vi "Lock in Amplifier.vi"() -> ()   [LabVIEW 2020]
uses:
  <vilib>/Utility/file.llb/Write Delimited Spreadsheet (DBL).vi
  Downloads/stanford_research_830/Stanford Research 830/Stanford Research 830.lvlib
panel:
  out "Waveform Graph":dynamicdata(graph)
  in  "Maximum Time (10000 ms)":u32=10000
  in  "Internal Reference Frequency (1000 Hz)":dbl=1000.0
  in  "Sine Output Amplitude (1 V)":dbl=1.0
  out "error out 2":errorcluster
  out "Measurements":sgl[](array[numeric])
  in  "Data Collection":T1={"Sample Rate (0: 62.5 mHz)"=0, "Continuous Storage (T: Enable)"=TRUE, "Number of Points (100)"=100, "Channel (1: Channel 1 Display)"=1, "Channel 1 Display (0: X)"=0} {"Channel 1 Display (0: X)" items=["X", "R", "X Noise", "Aux In 1", "Aux In 2"]; "Channel (1: Channel 1 Display)" items=["Channel 1 Display"=1, "Channel 2 Display"=2]; "Sample Rate (0: 62.5 mHz)" items=["62.5 mHz", "125 mHz", "250 mHz", "500 mHz", "1 Hz", "2 Hz", "4 Hz", "8Hz", "16 Hz", "32 Hz", "64 Hz", "128 Hz", "256 Hz", "512 Hz", "Trigger "]}
  in  "Configure":T2={"Lock in Amplifier PORT"="", "Input Connection (0: Single-Ended Voltage) "=0, "Input Coupling (0: AC)"=0, "Input Notch Filter (0: None)"=0, "Reference Source (1: Internal)"=1, "Dynamic Reserve (-1: Auto Reserve)"=-1, "Sensitivity (-1: Auto gain)"=-1, "Time Constant (8: 100ms)"=8} {"Time Constant (8: 100ms)" items=["10 us", "30 us", "100 us", "300 us", "1 ms", "3 ms", "10 ms", "30 ms", "100 ms", "300 ms", "1 s", "3 s", "10 s", "30 s", "100 s", "300 s", "1 ks", "3 ks", "10 ks", "30 ks"]; "Sensitivity (-1: Auto gain)" items=["Auto Gain"=-1, "2 nV/fA"=0, "5 nV/fA"=1, "10 nV/fA"=2, "20 nV/fA"=3, "50 nV/fA"=4, "100 nV/fA"=5, "200 nV/fA"=6, "500 nV/fA"=7, "1 uV/pA"=8, "2 uV/pA"=9, "5 uV/pA"=10, "10 uV/pA"=11, "20 uV/pA"=12, "50 uV/pA"=13, "100 uV/pA"=14, "200 uV/pA"=15, "500 uV/pA"=16, "1 mV/nA"=17, "2 mV/nA"=18, "5 mV/nA"=19, "10 mV/nA"=20, "20 mV/nA"=21, "50 mV/nA"=22, "100 mV/nA"=23, "200 mV/nA"=24, "500 mV/mA"=25, "1 V/uA"=26]; "Dynamic Reserve (-1: Auto Reserve)" items=["Auto Reserve"=-1, "High Reserve"=0, "Normal"=1, "Low Noise"=2]; "Reference Source (1: Internal)" items=["External", "Internal"]; "Input Notch Filter (0: None)" items=["None", "Line Notch", "2x Line Notch", "Both Notch Filters"]; "Input Coupling (0: AC)" items=["AC", "DC"]; "Input Connection (0: Single-Ended Voltage)" items=["Single-Ended Voltage", "Differential Voltage", "1 MOhm Current Gain", "100 MOhm Current Gain"]}
  out "error out":errorcluster
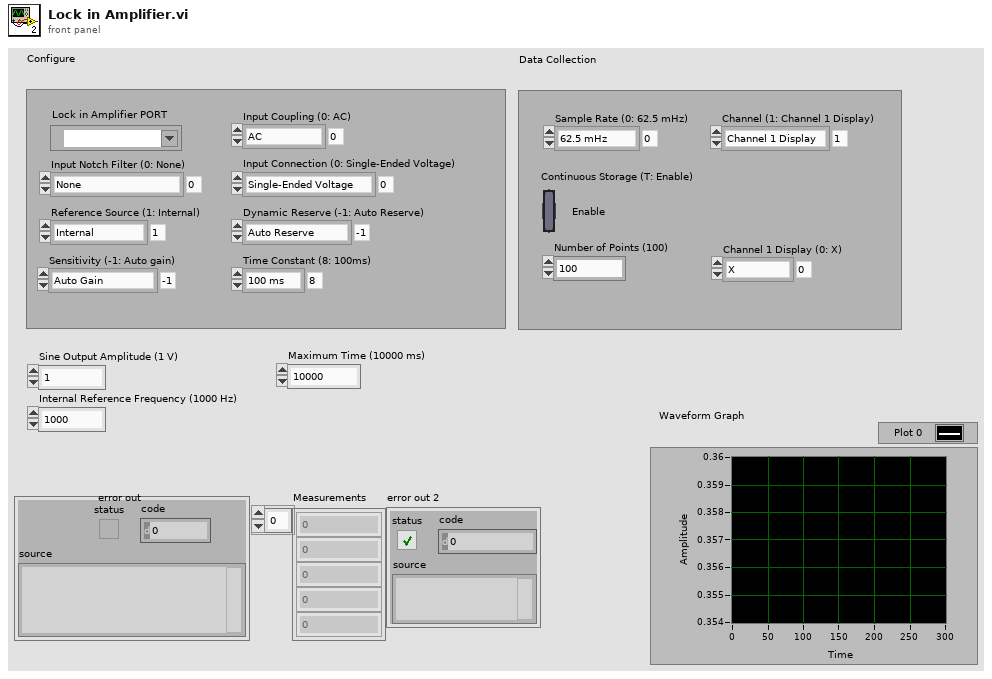
[diagram p1: front panel]
types:
  T1 = cluster{"Sample Rate (0: 62.5 mHz)":u16, "Continuous Storage (T: Enable)":bool, "Number of Points (100)":u32, "Channel (1: Channel 1 Display)":u16, "Channel 1 Display (0: X)":u16}
  T2 = cluster{"Lock in Amplifier PORT":refnum<visa-resource-name>, "Input Connection (0: Single-Ended Voltage) ":u16, "Input Coupling (0: AC)":u16, "Input Notch Filter (0: None)":u16, "Reference Source (1: Internal)":u16, "Dynamic Reserve (-1: Auto Reserve)":i16, "Sensitivity (-1: Auto gain)":i16, "Time Constant (8: 100ms)":u16}
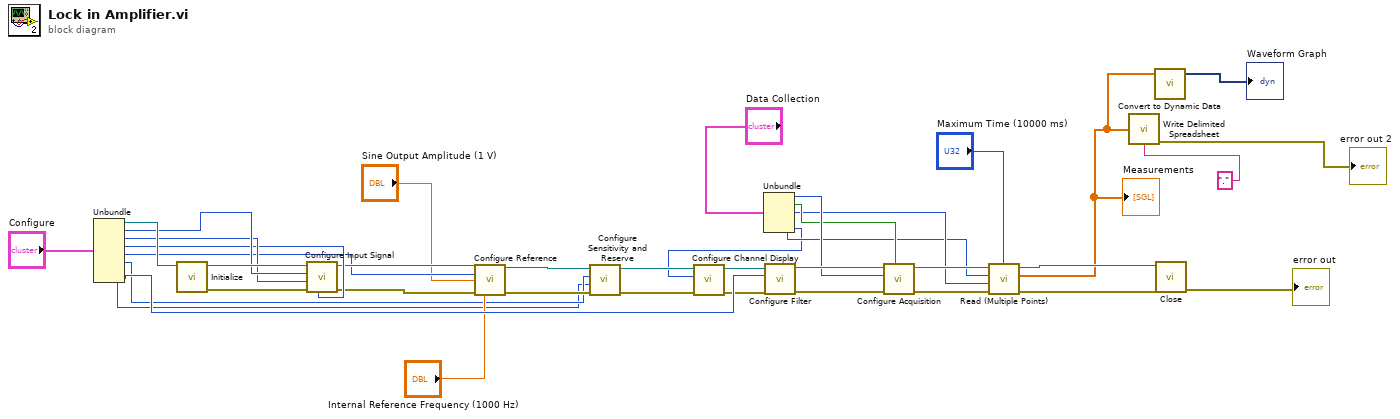
[diagram p0: block diagram]
diagram:
  n1 = Unbundle("Configure") -> ("Lock in Amplifier PORT"=w36:refnum<visa-resource-name>, "Input Connection (0: Single-Ended Voltage)"=w35:u16, "Input Coupling (0: AC)"=w34:u16, "Input Notch Filter (0: None)"=w33:u16, "Reference Source (1: Internal)"=w27:u16, "Dynamic Reserve (-1: Auto Reserve)"=w7:i16, "Sensitivity (-1: Auto gain)"=w6:i16, "Time Constant (8: 100ms)"=w25:u16)
  n2 = call "Initialize.vi"("VISA resource name"=w36) -> ("error out"=w38:errorcluster, "VISA resource name out"=w39:refnum<visa-resource-name>)  [unwired: 9 in]
  n3 = call "Configure Input Signal.vi"("Input Notch Filter (0: None)"=w33, "error in (no error)"=w38, "Input Coupling (0: AC)"=w34, "Input Connection (0: Single-Ended Voltage)"=w35, "VISA resource name"=w39) -> ("error out"=w26:errorcluster, "VISA resource name out"=w30:refnum<visa-resource-name>)  [unwired: 5 in]
  n4 = call "Configure Reference.vi"("VISA resource name"=w30, "Reference Source (1: Internal)"=w27, "Sine Output Amplitude (1 V)"="Sine Output Amplitude (1 V)", "error in (no error)"=w26, "Internal Reference Frequency (1000 Hz)"="Internal Reference Frequency (1000 Hz)") -> ("VISA resource name out"=w29:refnum<visa-resource-name>, "error out"=w28:errorcluster)  [unwired: 9 in]
  n5 = call "Configure Sensitivity and Reserve.vi"("error in (no error)"=w28, "Sensitivity (-1: Auto gain)"=w6, "Dynamic Reserve (-1: Auto Reserve)"=w7, "VISA resource name"=w29) -> ("error out"=w2:errorcluster, "VISA resource name out"=w3:refnum<visa-resource-name>)  [unwired: 6 in]
  n6 = Unbundle("Data Collection") -> ("Sample Rate (0: 62.5 mHz)"=w23:u16, "Continuous Storage (T: Enable)"=w22:bool, "Number of Points (100)"=w19:u32, "Channel (1: Channel 1 Display)"=w15:u16, "Channel 1 Display (0: X)"=w1:u16)
  n7 = call "Configure Channel Display.vi"("error in (no error)"=w2, "Channel 1 Display (0: X)"=w1, "VISA resource name"=w3) -> ("error out"=w4:errorcluster, "VISA resource name out"=w5:refnum<visa-resource-name>)  [unwired: 7 in]
  n8 = call "Configure Filter.vi"("error in (no error)"=w4, "Time Constant (8: 100ms)"=w25, "VISA resource name"=w5) -> ("error out"=w31:errorcluster, "VISA resource name out"=w32:refnum<visa-resource-name>)  [unwired: 7 in]
  n9 = call "Configure Acquisition.vi"("Continuous Storage (T: Enable)"=w22, "error in (no error)"=w31, "Sample Rate (0: 62.5 mHz)"=w23, "VISA resource name"=w32) -> ("error out"=w20:errorcluster, "VISA resource name out"=w21:refnum<visa-resource-name>)  [unwired: 6 in]
  n10 = call "Read (Multiple Points).vi"("Maximum Time (10000 ms)"="Maximum Time (10000 ms)", "error in (no error)"=w20, "Number of Points (100)"=w19, "Channel (1: Channel 1 Display)"=w15, "VISA resource name"=w21) -> ("error out"=w16:errorcluster, "Measurements"=w10:sgl[], "VISA resource name out"=w18:refnum<visa-resource-name>)  [unwired: 4 in]
  "Measurements" <- w10
  n11 = call-poly <vilib>:"Write Delimited Spreadsheet.vi"("1D data"=w10, "delimiter (\\t)"="." ("delimiter (\\t)")) -> ("error out"=→"error out 2":errorcluster)  [unwired: 12 in, 1 out]
  n12 = call "Convert to Dynamic Data"("Array"=w10) -> ("Dynamic Data Type"=→"Waveform Graph":dynamicdata)  [unwired: 3 in]
  n13 = call "Close.vi"("error in (no error)"=w16, "VISA resource name"=w18) -> ("error out"=→"error out":errorcluster)  [unwired: 9 in]
